vi "Process File.vi"(8 "error in (no error)":errorcluster, 10 "File":refnum<class "Acquired Result.lvclass">, 11 "Format Converter in":refnum<class "Format Converter.lvclass">) -> (0 "error out":errorcluster, 2 "File out":refnum<class "Acquired Result.lvclass">, 3 "Format Converter out":refnum<class "Format Converter.lvclass">)   [LabVIEW 2018, in "Format Converter.lvclass"]
uses:
  Format Converter.lvclass
  NHMFL_Core/Libraries/Instruments/Results/Acquired Result/Acquired Result.lvclass
  Read Format Converter Configuration.vi
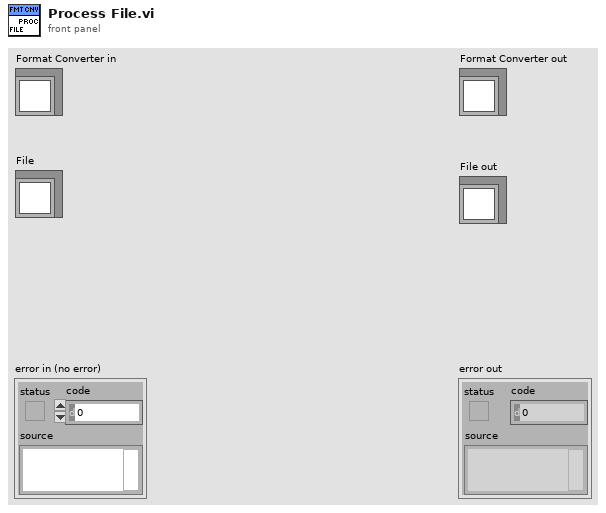
[diagram p1: front panel]
types:
  T1 = typedef "Format Converter Configuration.ctl" = cluster{"New start time":dbl, "New end time":dbl, "Output file format":enum16{"ASCII", "BINARY", "TDMS"}, "Save ASCII column names":bool, "Prepend binary array size":bool, "buffer size (-1: all)":i64, "Channels":string[], "Group":string, "New dt":dbl}
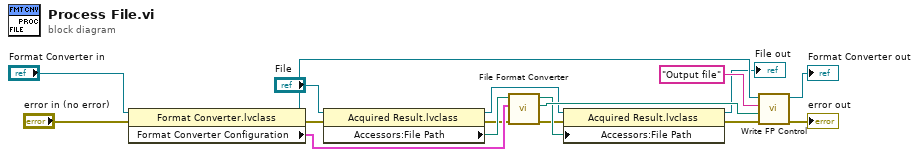
[diagram p0: block diagram]
diagram:
  n1 = property class="Format Converter.lvclass"(reference="Format Converter in", error in="error in (no error)") -> (reference out=w14:refnum<class "Format Converter.lvclass">, error out=w5:errorcluster, "Format Converter Configuration"=w16:T1)
  n2 = property class="Acquired Result.lvclass"(reference="File", error in=w5) -> (reference out=w7:refnum<class "Acquired Result.lvclass">, error out=w1:errorcluster, "Accessors:File Path"=w8:path)
  n3 = call "File Format Converter.vi"("Error In"=w1, "Configuration"=w16, "File"=w8) -> ("Error Out"=w4:errorcluster, "New file out"=w11:path, "File out"=w6:path)  [unwired: 6 in]
  n4 = property class="Acquired Result.lvclass"(reference=w7, error in=w4, "Accessors:File Path"=w6) -> (reference out=→"File out":refnum<class "Acquired Result.lvclass">, error out=w3:errorcluster)
  n5 = call-dynamic "Write FP Control.vi"("error in (no error)"=w3, "Control Value"=w11, "Control Name"="Output file", "Measure Object in"=w14) -> ("error out"=→"error out":errorcluster, "Measure Object out"=→"Format Converter out":refnum<class "Format Converter.lvclass">)  [unwired: 6 in]
